vi "AH 2700 Scan Measurement.vi"() -> ()   [LabVIEW 2019]
doc: "This example shows how to configure the bridge,initiate scan measurement, read the results from the bridge, and parse the measurement results."
uses:
  Andeen-Hagerling 2700(400 firmware).lvlib
panel:
  out "Attentap":string
  out "Loss Greater Than":string
  in  "Voltage Method":enum16{"discrete", "log10", "log2", "linear"}(ring)
  in  "Sample Method":enum16{"discrete"}(ring)
  in  "Frequency Method":enum16{"discrete", "log10", "log2", "linear"}(ring)
  in  "Voltage Method Value":dbl=1.0 min=-100.0 max=100.0 format="%#_6f"
  in  "Frequency Method Value":dbl=-12.0 min=-19000.0 max=19000.0
  in  "Total":i32 min=0 max=99999999
  in  "STMode":i32(ring) items=["Each", "Inner", "Second", "Third"]
  in  "Voltage Ceiling (V)":dbl=15.0 min=0.0003 max=15.0
  in  "Voltage Floor (V)":dbl=0.001 min=0.0003 max=15.0
  in  "Voltage Coupling":i32 min=0 max=3
  in  "Sample Method Value":i32(ring)=1 items=["-1"=-1, "1"=1]
  in  "Sample Ceiling":i32=8 min=1 max=8
  in  "Sample Floor":i32=1 min=1 max=8
  in  "Sample Coupling":i32 min=0 max=3
  in  "Frequency Ceiling (Hz)":dbl=20000.0 min=50.0 max=20000.0
  in  "Frequency Floor (Hz)":dbl=50.0 min=50.0 max=20000.0
  in  "Frequency Coupling":i32 min=0 max=3
  out "Loss Chart":dbl(graph)
  out "Capacitance Chart":dbl(graph)
  out "Sample Switch":i32
  in  "stop":bool
  out "Frequency (Hz)":dbl
  out "Units Display":i32(ring)=1 items=["nanosiemens"=1, "dissipation factor"=2, "kilohms"=3, "gigohms"=4, "loss vector (jpF)"=5]
  out "Error Message":string
  out "Voltage (V)":dbl format="%#_6f"
  out "Loss":dbl
  out "Capacitance (pF)":dbl format="%#_10f"
  in  "Units":i32(ring)=1 items=["nanosiemens"=1, "dissipation factor"=2, "kilohms"=3, "gigohms"=4, "loss vector (jpF)"=5]
  in  "Bridge Frequency (Hz)":dbl(ring)=1000.0 items=["50"=50.0, "60"=60.0, "70"=70.0, "80"=80.0, "100"=100.0, "120"=120.0, "140"=140.0, "160"=160.0, "200"=200.0, "240"=240.0, "300"=300.0, "400"=400.0, "500"=500.0, "600"=600.0, "700"=700.0, "800"=800.0, "1000"=1000.0, "1200"=1200.0, "1400"=1400.0, "1600"=1600.0, "2000"=2000.0, "2400"=2400.0, "3000"=3000.0, "4000"=4000.0, "5000"=5000.0, "6000"=6000.0, "7000"=7000.0, "8000"=8000.0, "10000"=10000.0, "12000"=12000.0, "14000"=14000.0, "16000"=16000.0, "20000"=20000.0]
  in  "Maximum Voltage (V)":dbl=15.0 min=0.0003 max=15.0 step=1.0 format="%#.6f"
  in  "Average Exponent":u16=4 max=15
  in  "VISA Resource":refnum<visa-resource-name>
  in  "Serial Configuration":T1={"Baud Rate"=9600, "Parity"=0, "Data Bits"=8, "Stop Bits"=10} {"Stop Bits" items=["1.0"=10, "1.5"=15, "2.0"=20]; "Data Bits" items=["7"=7, "8"=8]; "Parity" items=["None", "Odd", "Even", "Mark", "Space"]; "Baud Rate" items=["300"=300, "600"=600, "1200"=1200, "2400"=2400, "4800"=4800, "9600"=9600, "19200"=19200, "38400"=38400, "57600"=57600, "115200"=115200]}
  # "AH 2700A ULTRA-PRECISION 50Hz-20kHz CAPACITANCE BRIDGE"
  # "Scan Measurement"
  # "Measurement Parameters"
  # "Scan Parameters"
  # "Measurement Results"
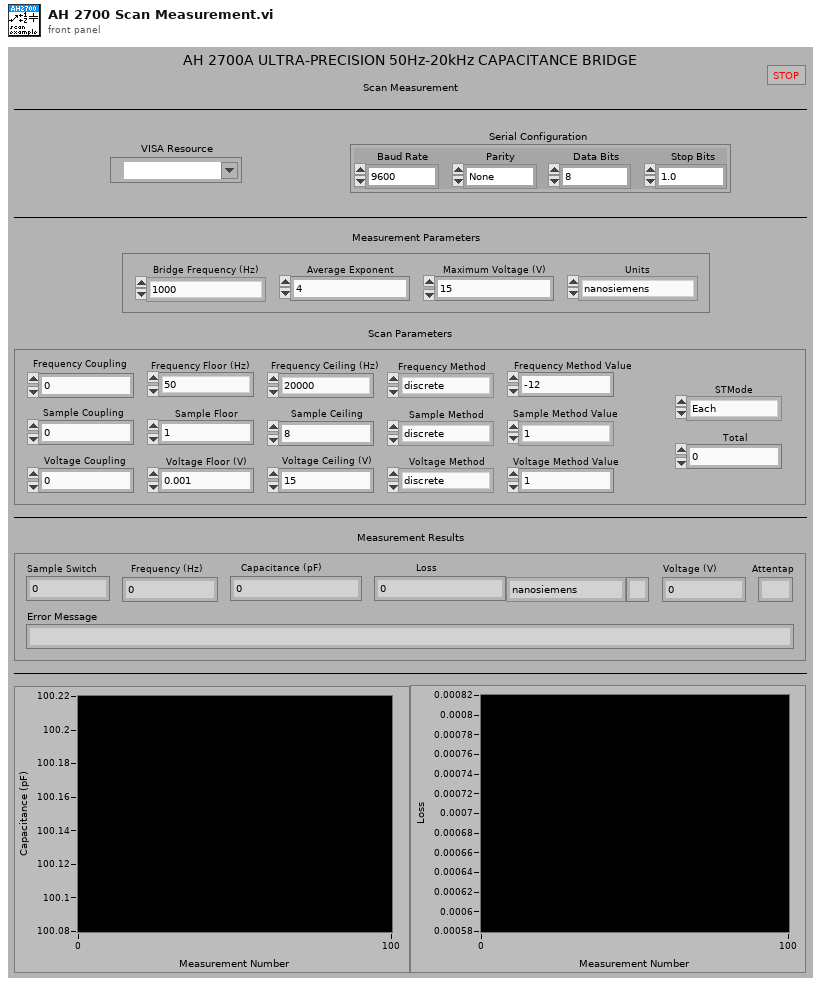
[diagram p1: front panel]
types:
  T1 = cluster{"Baud Rate":u32, "Parity":u16, "Data Bits":u16, "Stop Bits":u16}
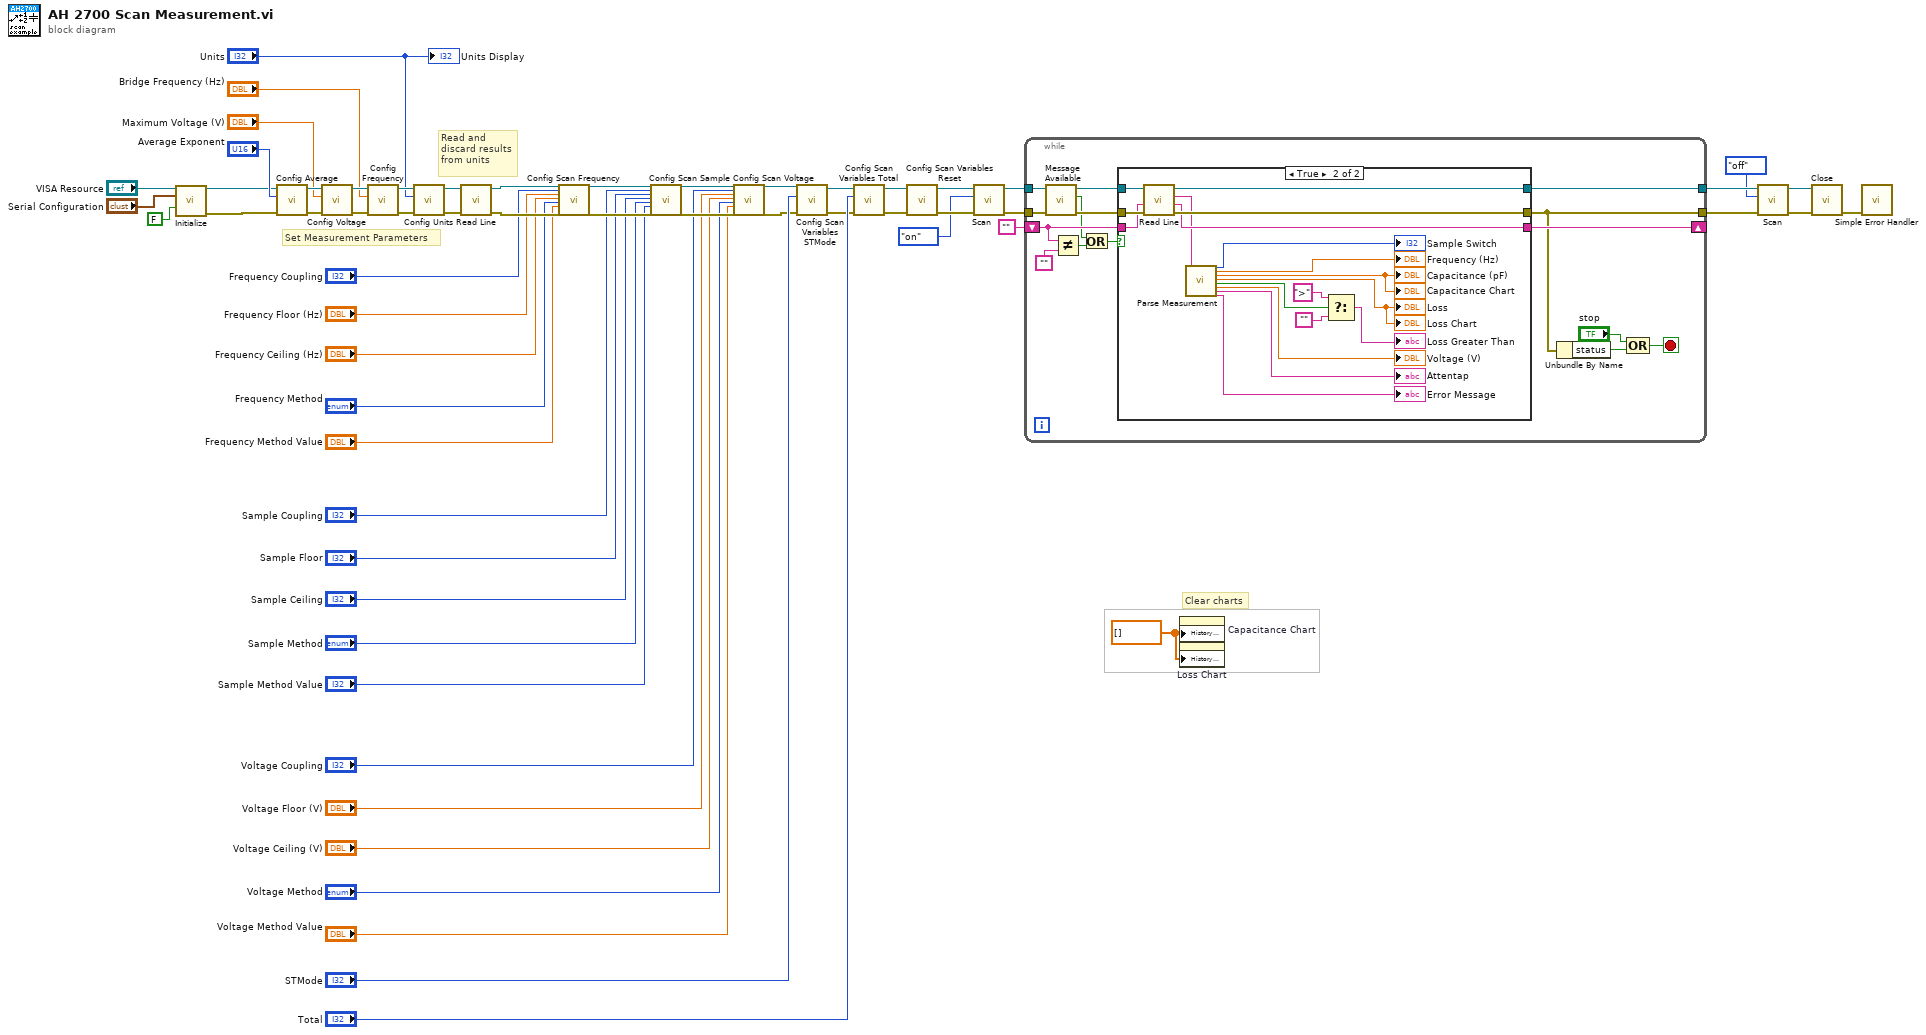
[diagram p0: block diagram]
diagram:
  w46 = dbl[] [] ("History Data")
  # "Clear charts"
  # "Set Measurement Parameters"
  # "Read and\ndiscard results\nfrom units"
  n1 = call "Initialize.vi"("VISA resource name"="VISA Resource", "Serial Configuration"="Serial Configuration", "Reset (True)"=FALSE) -> ("VISA resource name out"=w30:refnum<visa-resource-name>, "error out"=w29:errorcluster)  [unwired: 11 in]
  n2 = call "Config Average.vi"("error in"=w29, "Average Exponent (4)"="Average Exponent", "VISA resource name"=w30) -> ("error out"=w56:errorcluster, "VISA resource name out"=w59:refnum<visa-resource-name>)  [unwired: 7 in]
  n3 = call "Config Voltage.vi"("error in"=w56, "Voltage (15 V)"="Maximum Voltage (V)", "VISA resource name"=w59) -> ("error out"=w55:errorcluster, "VISA resource name out"=w58:refnum<visa-resource-name>)  [unwired: 7 in]
  n4 = call "Config Frequency.vi"("error in"=w55, "Frequency (1000 Hz)"="Bridge Frequency (Hz)", "VISA resource name"=w58) -> ("error out"=w54:errorcluster, "VISA resource name out"=w57:refnum<visa-resource-name>)  [unwired: 7 in]
  n5 = call "Config Units.vi"("error in"=w54, "Units (nS)"="Units", "VISA resource name"=w57) -> ("error out"=w49:errorcluster, "VISA resource name out"=w50:refnum<visa-resource-name>)  [unwired: 7 in]
  n6 = call "Read Line.vi"("error in"=w49, "VISA resource name"=w50) -> ("error out"=w25:errorcluster, "VISA resource name out"=w24:refnum<visa-resource-name>)  [unwired: 6 in, 2 out]
  n7 = call "Config Scan Frequency.vi"("VISA resource name"=w24, "Coupling (0)"="Frequency Coupling", "Floor (50 Hz)"="Frequency Floor (Hz)", "Ceiling (20000 Hz)"="Frequency Ceiling (Hz)", "Method (discrete)"="Frequency Method", "Method Value (-12)"="Frequency Method Value", "error in"=w25) -> ("VISA resource name out"=w18:refnum<visa-resource-name>, "error out"=w17:errorcluster)  [unwired: 19 in]
  n8 = call "Config Scan Sample.vi"("VISA resource name"=w18, "Coupling (0)"="Sample Coupling", "Floor (1)"="Sample Floor", "Ceiling (8)"="Sample Ceiling", "Method (discrete)"="Sample Method", "Method Value (1)"="Sample Method Value", "error in"=w17) -> ("VISA resource name out"=w11:refnum<visa-resource-name>, "error out"=w8:errorcluster)  [unwired: 19 in]
  n9 = call "Config Scan Voltage.vi"("VISA resource name"=w11, "Coupling (0)"="Voltage Coupling", "Floor (0.001)"="Voltage Floor (V)", "Ceiling (15)"="Voltage Ceiling (V)", "Method (discrete)"="Voltage Method", "Method Value (1)"="Voltage Method Value", "error in"=w8) -> ("VISA resource name out"=w10:refnum<visa-resource-name>, "error out"=w9:errorcluster)  [unwired: 19 in]
  n10 = call "Config Scan Variables STMode.vi"("error in"=w9, "Mode (Each)"="STMode", "VISA resource name"=w10) -> ("error out"=w32:errorcluster, "VISA resource name out"=w33:refnum<visa-resource-name>)  [unwired: 7 in]
  n11 = call "Config Scan Variables Total.vi"("error in"=w32, "Total (0)"="Total", "VISA resource name"=w33) -> ("error out"=w35:errorcluster, "VISA resource name out"=w37:refnum<visa-resource-name>)  [unwired: 7 in]
  n12 = call "Config Scan Variables Reset.vi"("error in"=w35, "VISA resource name"=w37) -> ("error out"=w34:errorcluster, "VISA resource name out"=w36:refnum<visa-resource-name>)  [unwired: 8 in]
  n13 = call "Scan.vi"("error in"=w34, "Scan Measurement (on)"=enum16{"off", "on"}."on", "VISA resource name"=w36) -> ("error out"=w39:errorcluster, "VISA resource name out"=w40:refnum<visa-resource-name>)  [unwired: 7 in]
  n14 = while {
    tunnel: [w66] -> w41
    tunnel: [w65] -> w43
    tunnel: w40 -> [w73]
    tunnel: w39 -> [w71]
    shift-right: [w74] -> _
    shift-left: "" -> [w64]
    stop <- w68 stop-if-true
    n15 = call "Message Available.vi"("error in"=w71, "VISA resource name"=w73) -> ("error out"=w70:errorcluster, "message available"=w61:bool, "VISA resource name out"=w72:refnum<visa-resource-name>)  [unwired: 7 in]
    n16 = Not Equal?(x=w64, y="") -> (x != y?=w62:bool)
    n17 = Or(x=w61, y=w62) -> (x .or. y?=w60:bool)
    n18 = case shown="True" w60 {
      tunnel: [w77 w95] -> w66
      tunnel: w72 -> [w77 w94]
      tunnel: w70 -> [w76 w93]
      tunnel: [w76 w92] -> w65
      tunnel: [w75 w90] -> w74
      tunnel: w64 -> [w75 w91]
      frame False {
      }
      frame True {
        n19 = call "Read Line.vi"("error in"=w93, "Previous"=w91, "VISA resource name"=w94) -> ("error out"=w92:errorcluster, "Remaining"=w90:string, "Message"=w89:string, "VISA resource name out"=w95:refnum<visa-resource-name>)  [unwired: 5 in]
        n20 = call "Parse Measurement.vi"("Measurement Line"=w89) -> ("Sample"=→"Sample Switch":i32, "Frequency"=→"Frequency (Hz)":dbl, "Capacitance"=→"Capacitance (pF)" →"Capacitance Chart":dbl, "Loss"=→"Loss" →"Loss Chart":dbl, "Loss Greater Than"=w84:bool, "Voltage"=→"Voltage (V)":dbl, "Attentap"=→"Attentap":string, "Error Message"=→"Error Message":string)  [unwired: 17 in, 2 out]
        n21 = Select(t=">", s=w84, f="") -> (s? t:f=→"Loss Greater Than":string)
      }
    }
    n22 = Unbundle By Name(w65) -> ("status"=w69:bool)
    n23 = Compound Arithmetic op=OR("stop", w69) -> (w68:bool)
  }
  n24 = property on="Capacitance Chart" class="WFChart (strict)"("History Data"=w46) -> ()  [unwired: 2 in, 2 out]
  n25 = property on="Loss Chart" class="WFChart (strict)"("History Data"=w46) -> ()  [unwired: 2 in, 2 out]
  n26 = call "Scan.vi"("error in"=w43, "Scan Measurement (on)"=enum16{"off", "on"}."off", "VISA resource name"=w41) -> ("error out"=w44:errorcluster, "VISA resource name out"=w42:refnum<visa-resource-name>)  [unwired: 7 in]
  n27 = call "Close.vi"("error in (no error)"=w44, "VISA resource name"=w42) -> ("error out"=w47:errorcluster)  [unwired: 9 in]
  n28 = call <vilib>:"Simple Error Handler.vi"("error in (no error)"=w47) -> ()  [unwired: 4 in, 5 out]
  "Units Display" <- "Units"
